vi "Create LVObjectMessage.vi"(8 "error in (no error)":errorcluster, 10 "Message Data":refnum<class>, 11 "Message Name":string) -> (0 "error out":errorcluster, 3 "LVObjectMessage out":refnum<class "LVObjectMessage.lvclass">)   [LabVIEW 2009, in "LapDog.Messaging.v2.NativeTypes.lvlib" / "LVObjectMessage.lvclass"]
doc: "Returns a LVObjectMessage object with the given name.\n\nThis method executes regardless of the error in state."
uses:
  LVObjectMessage.lvclass
  LVObjectMessage.lvclass/LVObjectMessage.ctl
  Messaging.v2/MessageObject/Message.lvclass
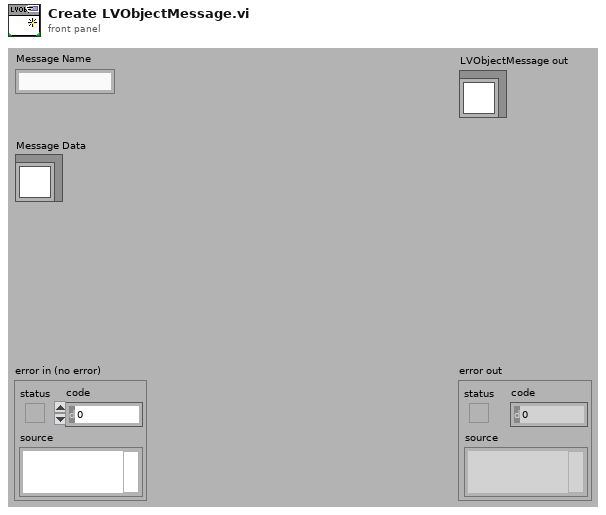
[diagram p1: front panel]
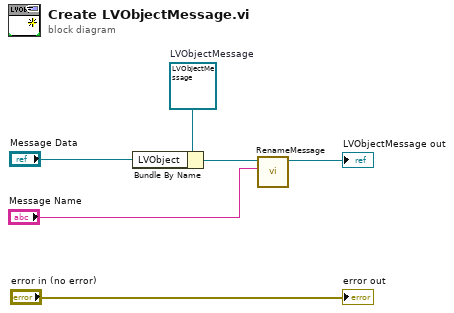
[diagram p0: block diagram]
diagram:
  w1 = refnum<class "LVObjectMessage.lvclass"> refnum  # LVObjectMessage
  n1 = Bundle By Name(cluster=w1, "LVObject"="Message Data") -> (w4:refnum<class "LVObjectMessage.lvclass">)
  n2 = call "RenameMessage.vi"("Message Name"="Message Name", "Message in"=w4) -> ("Message out"=→"LVObjectMessage out":refnum<class "LVObjectMessage.lvclass">)  [unwired: 8 in, 1 out]
  "error out" <- "error in (no error)"
